vi "Get Phasor Ratio.vi"(8 "Error In":errorcluster, 9 "Reference Phasor 2":T1, 10 "Reference Phasor 1":T1, 11 "Phasor":T1) -> (0 "Error Out":errorcluster, 3 "Phasor Ratio":dbl)   [LabVIEW 2019]
uses:
  Phasor (g, s).ctl
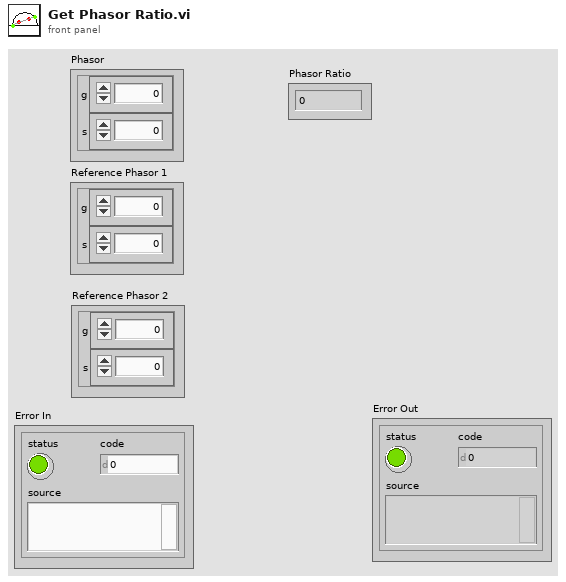
[diagram p1: front panel]
types:
  T1 = typedef "Phasor (g, s).ctl" = cluster{"g":dbl, "s":dbl}
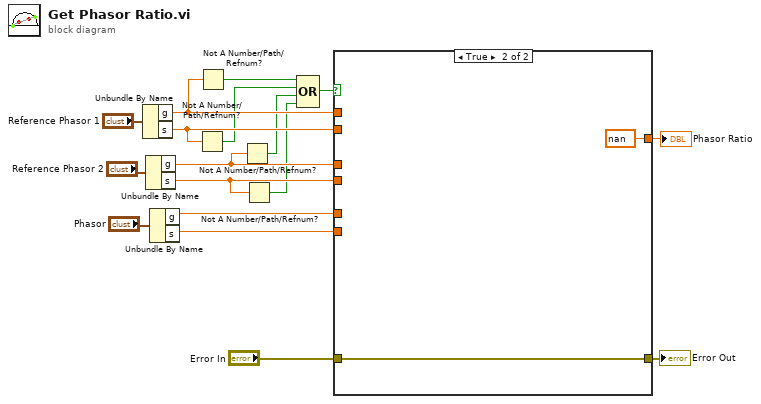
[diagram p0: block diagram]
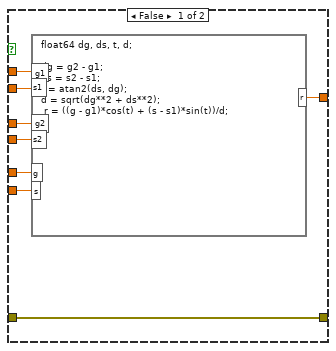
[diagram p2: hidden frame]
diagram:
  n1 = Unbundle By Name("Reference Phasor 1") -> ("g"=w11:dbl, "s"=w10:dbl)
  n2 = Unbundle By Name("Reference Phasor 2") -> ("g"=w9:dbl, "s"=w8:dbl)
  n3 = Unbundle By Name("Phasor") -> ("g"=w14:dbl, "s"=w13:dbl)
  n4 = Not A Number/Path/Refnum?(number/path/refnum=w10) -> (NaN/Path/Refnum?=w6:bool)
  n5 = Not A Number/Path/Refnum?(number/path/refnum=w11) -> (NaN/Path/Refnum?=w7:bool)
  n6 = Not A Number/Path/Refnum?(number/path/refnum=w9) -> (NaN/Path/Refnum?=w5:bool)
  n7 = Not A Number/Path/Refnum?(number/path/refnum=w8) -> (NaN/Path/Refnum?=w4:bool)
  n8 = Compound Arithmetic op=OR(w7, w6, w5, w4) -> (w3:bool)
  n9 = case shown="True" w3 {
    tunnel: w14 -> [w25 _]
    tunnel: w13 -> [w24 _]
    tunnel: [w23 nan ("r")] -> w12
    tunnel: w11 -> [w22 _]
    tunnel: w10 -> [w21 _]
    tunnel: w9 -> [w20 _]
    tunnel: w8 -> [w19 _]
    tunnel: "Error In" -> [w18 w26]
    tunnel: [w18 w26] -> w1
    frame False {
      n10 = formula code="float64 dg, ds, t, d;\n\ndg = g2 - g1;\nds = s2 - s1;\nt = atan2(ds, dg);\nd = sqrt(dg**2 + ds**2);\n r = ((g - g1)*cos(t) + (s - s1)*sin(t))/d;"("g1"=w22, "s1"=w21, "g2"=w20, "s2"=w19, "g"=w25, "s"=w24) -> ("r"=w23:dbl)
    }
    frame True {
    }
  }
  "Phasor Ratio" <- w12
  "Error Out" <- w1
